vi "Word_Insert_Text_(str).vi"(0 "Word._Document":refnum<k7>, 1 "font":T1 {"font size" format="%.2f"; "strike through" items=["Unchanged", "Yes", "No"]; "underline" items=["Unchanged", "Yes", "No"]; "italic" items=["Unchanged", "Yes", "No"]; "bold" items=["Unchanged", "Yes", "No"]}, 2 "Style":string, 3 "from template?":bool, 5 "Text":string, 7 "Start":i32, 9 "End":i32, 11 "Error in (no error)":errorcluster, 12 "Insertion point":u16(ring)=1 items=["begining of document", "end of document", "bookmark", "custom"], 13 "Bookmark name":string) -> (4 "ActiveDocument out":refnum<k7>, 8 "Start out":i32, 10 "End out":i32, 15 "Error out":errorcluster={"status"=FALSE, "code"=0, "source"=" "})   [LabVIEW 2020, in "NI_ReportGenerationToolkit.lvlib"]
uses:
  <vilib>/addons/_office/NI_ReportGenerationToolkit.lvlib
  <vilib>/addons/_office/_exclsub.llb/font.ctl
panel:
  # "Content"
  # "Position"
  # "Output"
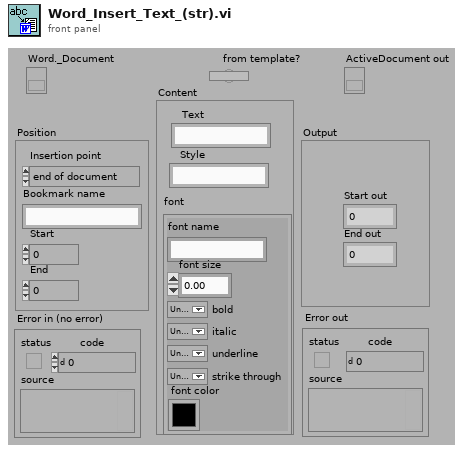
[diagram p1: front panel]
types:
  T1 = typedef "NI_ReportGenerationToolkit.lvlib/font.ctl" = cluster{"font name":string, "font size":dbl, "bold":u16, "italic":u16, "underline":u16, "strike through":u16, "font color":u32}
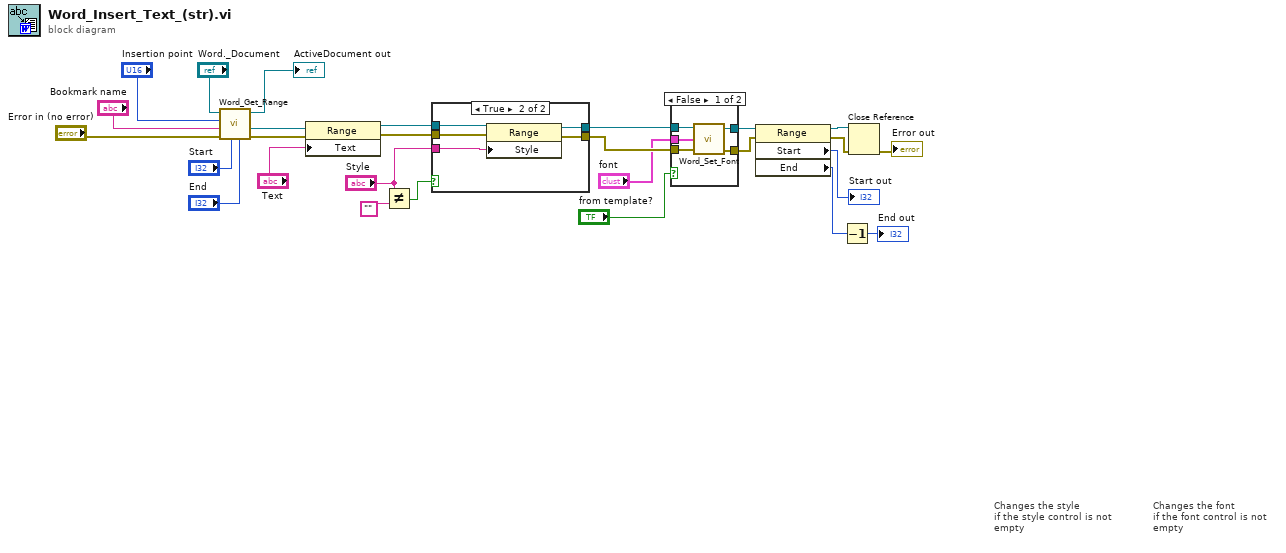
[diagram p0: block diagram]
diagram:
  # "Changes the font\nif the font control is not\nempty"
  # "Changes the style\nif the style control is not\nempty"
  n1 = call <vilib>:"Word_Get_Range.vi"("end"="End", "start"="Start", "error in"="Error in (no error)", "bookmark name"="Bookmark name", "insertion point"="Insertion point", "document in"="Word._Document") -> ("error out (no error)"=w21:errorcluster, "range"=w20:refnum<k7>, "document out"=→"ActiveDocument out":refnum<k7>)  [unwired: 3 out]
  n2 = property class="Range"(reference=w20, error in=w21, "Text"="Text") -> (reference out=w11:refnum<k7>, error out=w10:errorcluster)
  n3 = Not Equal?(x="Style", y="") -> (x != y?=w6:bool)
  n4 = case shown="True" w6 {
    tunnel: w11 -> [w29 w34]
    tunnel: w10 -> [w28 w33]
    tunnel: [w29 w32] -> w9
    tunnel: [w28 w31] -> w8
    tunnel: "Style" -> [_ w30]
    frame False {
    }
    frame True {
      n5 = property class="Range"(reference=w34, error in=w33, "Style"=w30) -> (reference out=w32:refnum<k7>, error out=w31:errorcluster)
    }
  }
  n6 = case shown="False" "from template?" {
    tunnel: [w39 w41] -> w19
    tunnel: [w38 w40] -> w17
    tunnel: w9 -> [w37 w41]
    tunnel: w8 -> [w36 w40]
    tunnel: "font" -> [w35 _]
    frame False {
      n7 = call <vilib>:"Word_Set_Font.vi"("Range in"=w37, "font"=w35, "Error in"=w36) -> ("Range out"=w39:refnum<k7>, "Error out"=w38:errorcluster)  [unwired: 5 out]
    }
    frame True {
    }
  }
  n8 = property class="Range"(reference=w19, error in=w17) -> (reference out=w18:refnum<k7>, error out=w16:errorcluster, "Start"=→"Start out":i32, "End"=w14:i32)
  n9 = Decrement(x=w14) -> (x-1=→"End out":i32)
  n10 = Close Reference(reference=w18, error in (no error)=w16) -> (error out=→"Error out":errorcluster)
